vi "Conversion Options.vi"(8 "Save a copy of the Binary Data File":bool=TRUE) -> (0 "Save Each Channel as a Separate File indicator":bool, 3 "Array":bool[](array[boolean]), 4 "Save a copy of the Binary Data File":bool)   [LabVIEW 2023]
panel:
  in  "dt (s)":bool=TRUE
  in  "All On":bool
  in  "All Off":bool
  in  "Save":bool
  in  "Save Each Channel as a Separate File":bool
  in  "FeedbackT":bool=TRUE
  in  "Line Num":bool=TRUE
  in  "C2":bool=TRUE
  in  "Phase":bool=TRUE
  in  "Amp":bool=TRUE
  in  "C3":bool=TRUE
  in  "C1":bool=TRUE
  in  "V2":bool=TRUE
  in  "V":bool=TRUE
  in  "Z":bool=TRUE
  in  "Y":bool=TRUE
  in  "X":bool=TRUE
  # "Channels to convert"
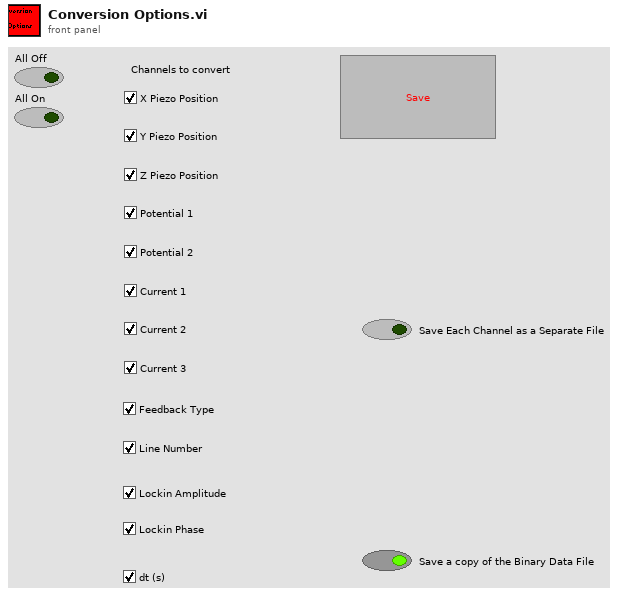
[diagram p1: front panel]
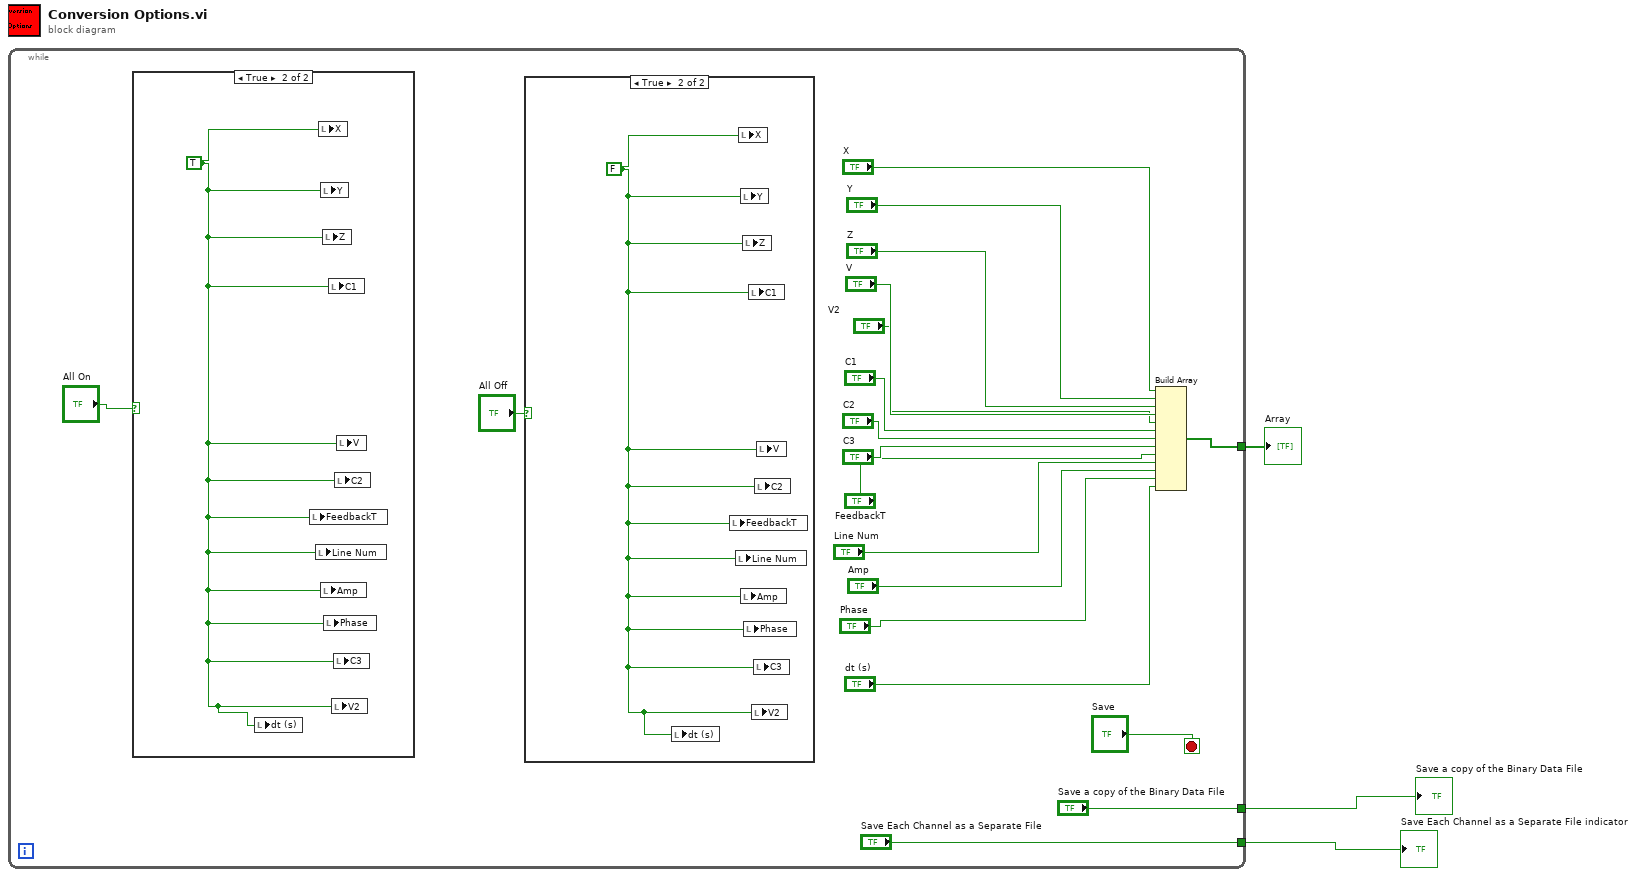
[diagram p0: block diagram]
diagram:
  n1 = while {
    tunnel: ["Save Each Channel as a Separate File"] -> w3
    tunnel: [w20] -> w1
    tunnel: ["Save a copy of the Binary Data File"] -> w2
    stop <- "Save" stop-if-true
    n2 = case shown="True" "All On" {
      frame False {
      }
      frame True {
        w24 = TRUE
        n3 = local write "dt (s)"(w24) -> ()
        n4 = local write "FeedbackT"(w24) -> ()
        n5 = local write "Line Num"(w24) -> ()
        n6 = local write "X"(w24) -> ()
        n7 = local write "Y"(w24) -> ()
        n8 = local write "Amp"(w24) -> ()
        n9 = local write "Z"(w24) -> ()
        n10 = local write "Phase"(w24) -> ()
        n11 = local write "C1"(w24) -> ()
        n12 = local write "V2"(w24) -> ()
        n13 = local write "C3"(w24) -> ()
        n14 = local write "C2"(w24) -> ()
        n15 = local write "V"(w24) -> ()
      }
    }
    n16 = case shown="True" "All Off" {
      frame False {
      }
      frame True {
        w23 = FALSE
        n17 = local write "dt (s)"(w23) -> ()
        n18 = local write "FeedbackT"(w23) -> ()
        n19 = local write "Line Num"(w23) -> ()
        n20 = local write "X"(w23) -> ()
        n21 = local write "Y"(w23) -> ()
        n22 = local write "Amp"(w23) -> ()
        n23 = local write "Z"(w23) -> ()
        n24 = local write "Phase"(w23) -> ()
        n25 = local write "C1"(w23) -> ()
        n26 = local write "V2"(w23) -> ()
        n27 = local write "C3"(w23) -> ()
        n28 = local write "C2"(w23) -> ()
        n29 = local write "V"(w23) -> ()
      }
    }
    n30 = Build Array("X", "Y", "Z", "V", "V2", "C1", "C2", "C3", "FeedbackT", "Line Num", "Amp", "Phase", "dt (s)") -> (w20:bool[])
  }
  "Save Each Channel as a Separate File indicator" <- w3
  "Array" <- w1
  "Save a copy of the Binary Data File" <- w2
